vi "Robot Systems.vi"(11 "input cluster":T1) -> ()   [LabVIEW 2015]
uses:
  Joystick/ControlsToCommands.ctl
  Robot Global Data.vi
panel:
  in  "Keep Vis Run":bool
  in  "Power":dbl=1.0
  out "What to do 2nd":string
  out "What to do 1st":string
  in  "Speed In":dbl=0.14
  in  "Time In":dbl=0.25
  in  "Vis Run":bool
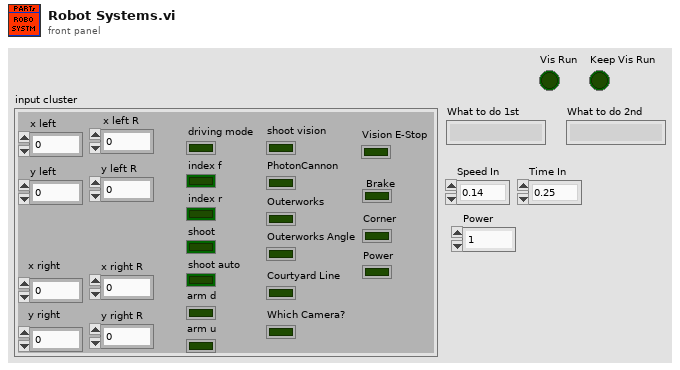
[diagram p1: front panel]
types:
  T1 = typedef "ControlsToCommands.ctl" = cluster{"x left":dbl, "y left":dbl, "x right":dbl, "y right":dbl, "driving mode":bool, "index f":bool, "index r":bool, "shoot":bool, "shoot auto":bool, "arm d":bool, "arm u":bool, "shoot vision":bool, "PhotonCannon":bool, "Outerworks":bool, "Outerworks Angle":bool, "Courtyard Line":bool, "Which Camera?":bool, "Vision E-Stop":bool, "x left R":dbl, "y left R":dbl, "x right R":dbl, "y right R":dbl, "Brake":bool, "Corner":bool, "Power":bool}
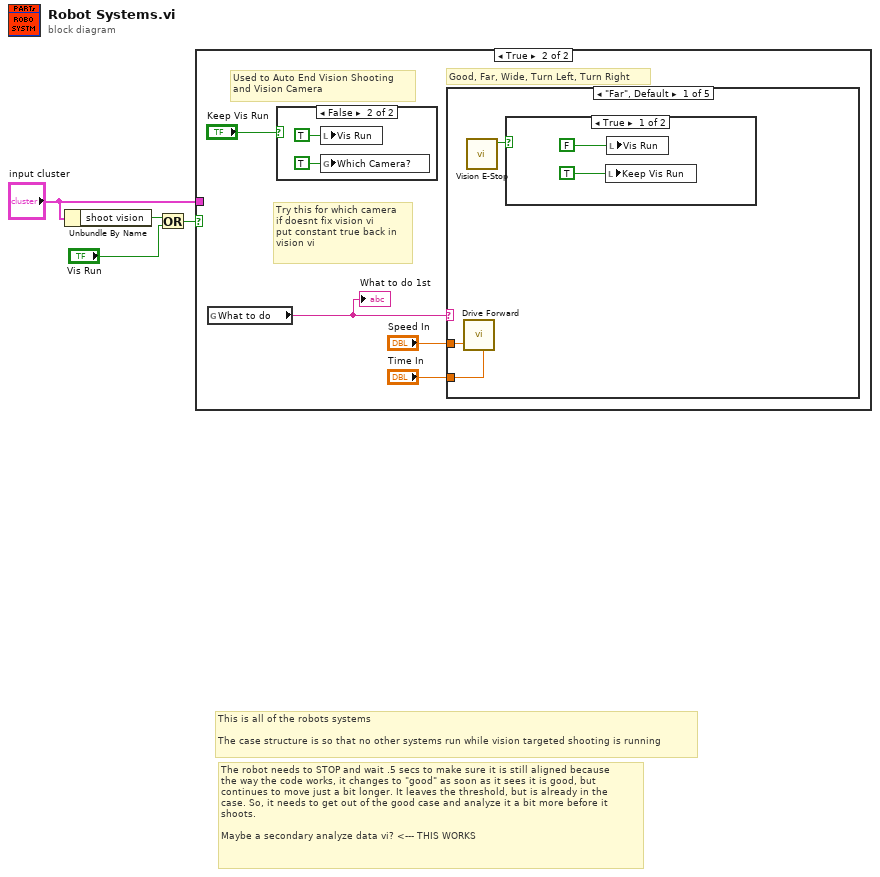
[diagram p0: block diagram]
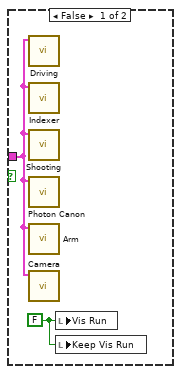
[diagram p2: hidden frame]
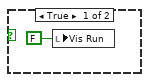
[diagram p3: hidden frame]
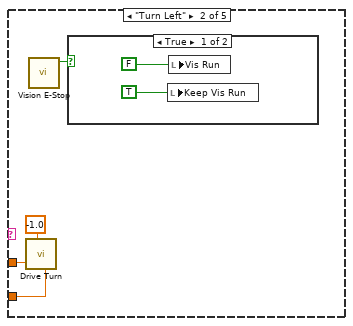
[diagram p5: hidden frame]
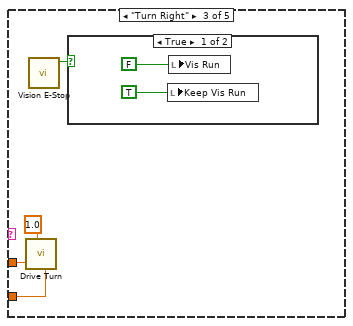
[diagram p7: hidden frame]
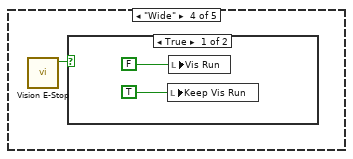
[diagram p9: hidden frame]
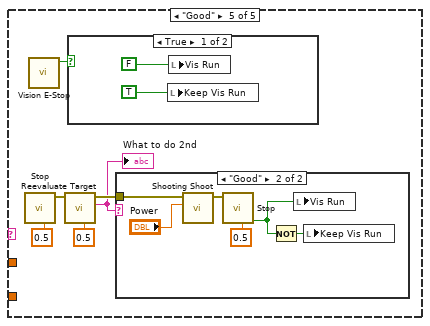
[diagram p11: hidden frame]
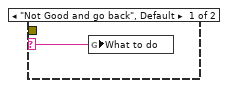
[diagram p13: hidden frame]
diagram:
  # "The robot needs to STOP and wait .5 secs to make sure it is still aligned because \nthe way the code works, it changes to \"good\" as soon as it sees it is good, but \ncontinues to move just a bit longer. It leaves the threshold, but is already in the \ncase. So, it needs to get out of the good case and analyze it a bit more before it \nshoots.\n\nMaybe a secondary analyze data vi? <--- THIS WORKS"
  # "This is all of the robots systems\n\nThe case structure is so that no other systems run while vision targeted shooting is running"
  n1 = Unbundle By Name("input cluster") -> ("shoot vision"=w2:bool)
  n2 = Or(x=w2, y="Vis Run") -> (x .or. y?=w3:bool)
  n3 = case shown="True" w3 {
    tunnel: "input cluster" -> [w6 _]
    frame False {
      w5 = FALSE ("Vision Running")
      n4 = call "Driving.vi"("input cluster"=w6) -> ()  [unwired: 11 in]
      n5 = call "Indexer.vi"("input cluster"=w6) -> ()  [unwired: 11 in]
      n6 = call "Shooting.vi"("input cluster"=w6) -> ()  [unwired: 11 in]
      n7 = call "Photon Canon.vi"("input cluster"=w6) -> ()  [unwired: 11 in]
      n8 = call "Arm.vi"("input cluster"=w6) -> ()  [unwired: 11 in]
      n9 = call "Camera.vi"("input cluster"=w6) -> ()  [unwired: 11 in]
      n10 = local write "Vis Run"(w5) -> ()
      n11 = local write "Keep Vis Run"(w5) -> ()
    }
    frame True {
      # "Try this for which camera\nif doesnt fix vision vi\nput constant true back in \nvision vi"
      # "Good, Far, Wide, Turn Left, Turn Right"
      # "Used to Auto End Vision Shooting \nand Vision Camera"
      n12 = global read "Robot Global Data.vi" "What to do"() -> (w7:string)
      "What to do 1st" <- w7
      n13 = case shown="False" "Keep Vis Run" {
        frame True {
          n14 = local write "Vis Run"(FALSE ("Done")) -> ()
        }
        frame False {
          n15 = local write "Vis Run"(TRUE ("Done")) -> ()
          n16 = global write "Robot Global Data.vi" "Which Camera?"(TRUE ("Which Camera?")) -> ()
        }
      }
      n17 = case shown="\"Far\", Default" w7 {
        tunnel: "Speed In" -> [w16 w21 w27 _ _]
        tunnel: "Time In" -> [w15 w20 w26 _ _]
        frame "Far", Default {
          n18 = call "Drive Forward.vi"("Time"=w15, "Speed"=w16) -> ()  [unwired: 9 in, 1 out]
          n19 = call "Vision E-Stop.vi"() -> ("E-Stop"=w14:bool)  [unwired: 11 in]
          n20 = case shown="True" w14 {
            frame True {
              n21 = local write "Keep Vis Run"(TRUE ("Done")) -> ()
              n22 = local write "Vis Run"(FALSE ("Done")) -> ()
            }
            frame False {
            }
          }
        }
        frame "Turn Left" {
          n23 = call "Drive Turn.vi"("Time"=w20, "Speed"=w21, "Direction"=-1.0) -> ()  [unwired: 8 in, 1 out]
          n24 = call "Vision E-Stop.vi"() -> ("E-Stop"=w22:bool)  [unwired: 11 in]
          n25 = case shown="True" w22 {
            frame True {
              n26 = local write "Keep Vis Run"(TRUE ("Done")) -> ()
              n27 = local write "Vis Run"(FALSE ("Done")) -> ()
            }
            frame False {
            }
          }
        }
        frame "Turn Right" {
          n28 = call "Drive Turn.vi"("Time"=w26, "Speed"=w27, "Direction"=1.0) -> ()  [unwired: 8 in, 1 out]
          n29 = call "Vision E-Stop.vi"() -> ("E-Stop"=w28:bool)  [unwired: 11 in]
          n30 = case shown="True" w28 {
            frame True {
              n31 = local write "Keep Vis Run"(TRUE ("Done")) -> ()
              n32 = local write "Vis Run"(FALSE ("Done")) -> ()
            }
            frame False {
            }
          }
        }
        frame "Wide" {
          n33 = call "Vision E-Stop.vi"() -> ("E-Stop"=w31:bool)  [unwired: 11 in]
          n34 = case shown="True" w31 {
            frame True {
              n35 = local write "Keep Vis Run"(TRUE ("Done")) -> ()
              n36 = local write "Vis Run"(FALSE ("Done")) -> ()
            }
            frame False {
            }
          }
        }
        frame "Good" {
          n37 = call "Stop.vi"("Time"=0.5) -> ("error out"=w38:errorcluster)  [unwired: 9 in, 1 out]
          n38 = call "Vision E-Stop.vi"() -> ("E-Stop"=w34:bool)  [unwired: 11 in]
          n39 = call "Reevaluate Target.vi"("Delay Time (s)"=0.5 ("Time"), "error in (no error)"=w38) -> ("What to do"=w35:string, "error out (no error)"=w36:errorcluster)  [unwired: 8 in]
          "What to do 2nd" <- w35
          n40 = case shown="True" w34 {
            frame True {
              n41 = local write "Keep Vis Run"(TRUE ("Done")) -> ()
              n42 = local write "Vis Run"(FALSE ("Done")) -> ()
            }
            frame False {
            }
          }
          n43 = case shown="\"Good\"" w35 {
            selector: w35 -> [w42 _]
            tunnel: w36 -> [_ w48]
            frame "Not Good and go back", Default {
              n44 = global write "Robot Global Data.vi" "What to do"(w42) -> ()
            }
            frame "Good" {
              n45 = call "Shooting Shoot.vi"("Power"="Power", "error in (no error)"=w48) -> ("error out"=w46:errorcluster)  [unwired: 9 in]
              n46 = call "Stop.vi"("Time"=0.5, "error in"=w46) -> ("Done"=w44:bool)  [unwired: 8 in, 1 out]
              n47 = Not(x=w44) -> (.not. x?=w45:bool)
              n48 = local write "Vis Run"(w44) -> ()
              n49 = local write "Keep Vis Run"(w45) -> ()
            }
          }
        }
      }
    }
  }
